vi "Initialize.vi"(7 "Serial Configuration":T1={"Baud Rate"=9600, "Parity"=2, "Data Bits"=7, "Stop Bits"=10, "Flow Control"=0} {"Flow Control" items=["None", "XON/XOFF", "RTS/CTS", "XON/XOFF & RTS/CTS", "DTR/DSR", "XON/XOFF & DTR/DSR"]; "Stop Bits" items=["1.0"=10, "1.5"=15, "2.0"=20]; "Data Bits" items=["7"=7, "8"=8]; "Parity" items=["None", "Odd", "Even", "Mark", "Space"]; "Baud Rate" items=["300"=300, "600"=600, "1200"=1200, "2400"=2400, "4800"=4800, "9600"=9600, "19200"=19200]}, 8 "error in (no error)":errorcluster, 10 "ID Query (False)":bool, 11 "VISA resource name":refnum<visa-resource-name>) -> (0 "error out":errorcluster, 3 "VISA resource name out":refnum<visa-resource-name>)   [LabVIEW 2018]
doc: "Establishes communication with the instrument and optionally performs an instrument identification query and/or an instrument reset. It also places the instrument in a default state needed for other instrument driver operations. Therefore, call this VI before calling other instrument driver VIs for this instrument. Generally, you need to call the <b>Initialize</b> VI only once at the beginning of an application."
panel:
  # "(c) 2014 <Enter Company Name Here>.  ALL RIGHTS RESERVED."
  # "EDIT: Change control description to remove example text for buses not supported."
  # "EDIT: Serial settings must match those on the physical instrument.  Review user's manual to determine the correct Flow Control protocol for the instrument.  \"None\" is the least robust option for this setting, and could lead to unreliable data transmission."
  # "EDIT: If your instrument does not support ID query or Reset, remove the ID Query or Reset control from the front panel and delete the case structure with the ID Query or Reset code from the block diagram."
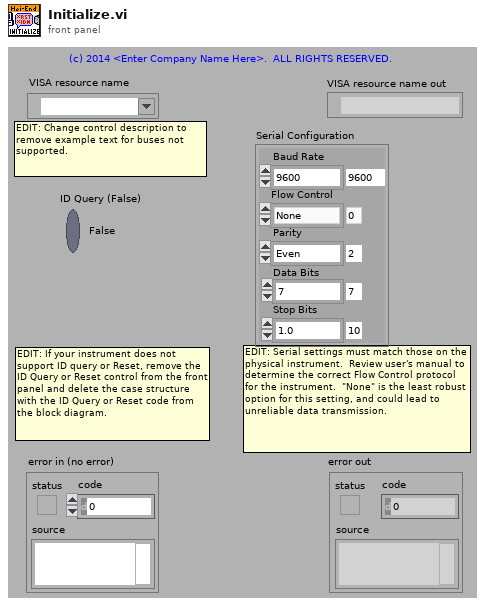
[diagram p1: front panel]
types:
  T1 = cluster{"Baud Rate":u32, "Parity":u16, "Data Bits":u16, "Stop Bits":u16, "Flow Control":u16}
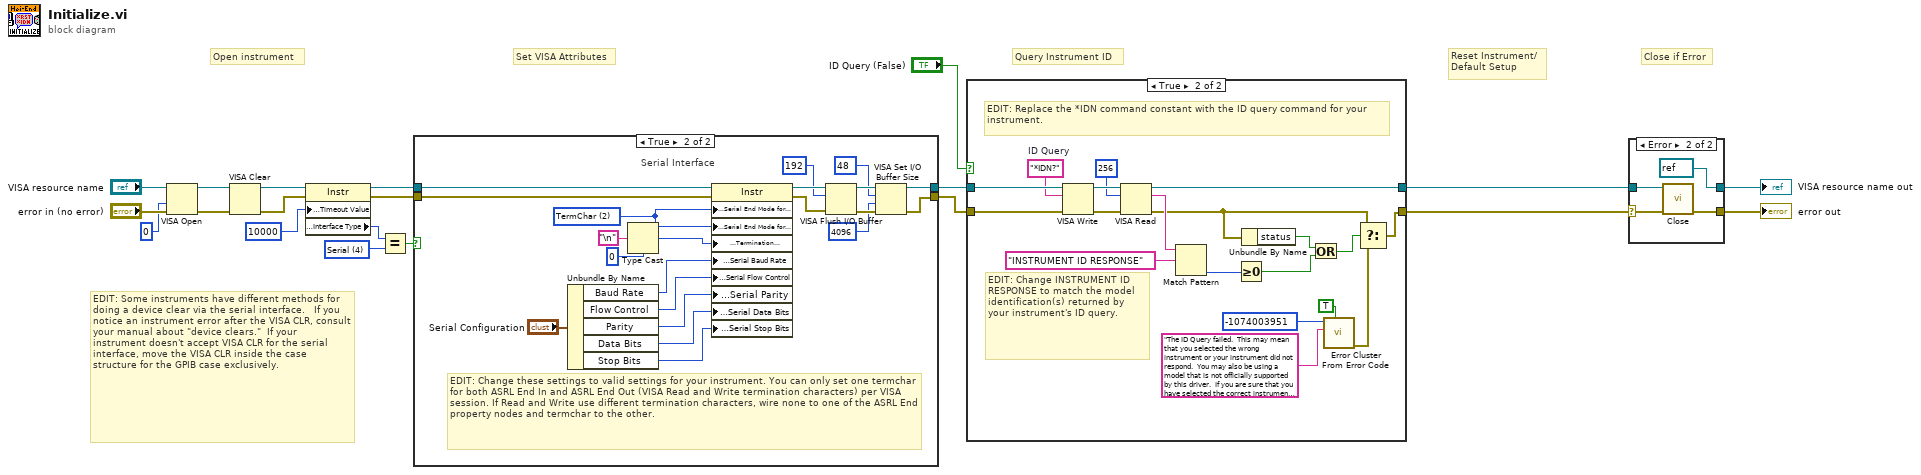
[diagram p0: block diagram]
diagram:
  w10 = u16 4 items=["GPIB"=1, "VXI"=2, "GPIB-VXI"=3, "Serial"=4, "PXI"=5, "TCPIP"=6, "USB"=7] ("Interface Information:Interface Type")
  # "EDIT: Some instruments have different methods for doing a device clear via the serial interface.   If you notice an instrument error after the VISA CLR, consult your manual about \"device clears.\"  If your instrument doesn't accept VISA CLR for the serial interface, move the VISA CLR inside the case  structure for the GPIB case exclusively."
  # "Set VISA Attributes"
  # "Close if Error"
  # "Query Instrument ID"
  # "Reset Instrument/\nDefault Setup"
  # "Open instrument"
  n1 = VISA Open(access mode=u32 0, error in (no error)="error in (no error)", VISA resource name="VISA resource name") -> (VISA resource name=w8:refnum<visa-resource-name>, error out=w7:errorcluster)  [unwired: 2 in]
  n2 = VISA Clear(VISA resource name=w8, error in (no error)=w7) -> (VISA resource name out=w6:refnum<visa-resource-name>, error out=w5:errorcluster)
  n3 = property class="Instr"(reference=w6, error in=w5, "General Settings:Timeout Value"=u32 10000) -> (reference out=w13:refnum<visa-resource-name>, error out=w12:errorcluster, "Interface Information:Interface Type"=w17:u16)
  n4 = Equal?(x=w17, y=w10) -> (x = y?=w11:bool)
  n5 = case shown="True" w11 {
    tunnel: [w21 w40] -> w15
    tunnel: [w22 w37] -> w14
    tunnel: w13 -> [w21 w42]
    tunnel: w12 -> [w22 w43]
    frame False {
      # "EDIT: Remove interfaces not supported by your instrument."
      # "GPIB, TCP/IP, and USB Interface"
    }
    frame True {
      w30 = u16 2 items=["None", "LastBit", "TermChar"] ("Serial Settings:Serial End Mode for Reads")
      # "EDIT: Change these settings to valid settings for your instrument. You can only set one termchar for both ASRL End In and ASRL End Out (VISA Read and Write termination characters) per VISA session. If Read and Write use different termination characters, wire none to one of the ASRL End property nodes and termchar to the other."
      # "Serial Interface"
      n6 = Unbundle By Name("Serial Configuration") -> ("Baud Rate"=w28:u32, "Flow Control"=w24:u16, "Parity"=w26:u16, "Data Bits"=w27:u16, "Stop Bits"=w23:u16)
      n7 = Type Cast(type=u8 0, x="\n" ("Line Feed Constant")) -> (*(type *) &x=w29:u8)
      n8 = property class="Instr"(reference=w42, error in=w43, "Serial Settings:Serial End Mode for Reads"=w30, "Serial Settings:Serial End Mode for Writes"=w30, "Message Based Settings:Termination Character"=w29, "Serial Settings:Serial Baud Rate"=w28, "Serial Settings:Serial Flow Control"=w24, "Serial Settings:Serial Parity"=w26, "Serial Settings:Serial Data Bits"=w27, "Serial Settings:Serial Stop Bits"=w23) -> (reference out=w36:refnum<visa-resource-name>, error out=w39:errorcluster)
      n9 = VISA Flush I/O Buffer(VISA resource name=w36, mask (16)=u16 192, error in (no error)=w39) -> (VISA resource name out=w41:refnum<visa-resource-name>, error out=w38:errorcluster)
      n10 = VISA Set I/O Buffer Size(VISA resource name=w41, mask (16)=u16 48, size (4096)=u32 4096 ("size (0)"), error in (no error)=w38) -> (VISA resource name out=w40:refnum<visa-resource-name>, error out=w37:errorcluster)
    }
  }
  n11 = case shown="True" "ID Query (False)" {
    tunnel: [w44 w64] -> w1
    tunnel: [w45 w61] -> w2
    tunnel: w15 -> [w45 w62]
    tunnel: w14 -> [w44 w63]
    frame False {
    }
    frame True {
      w55 = "*IDN?"  # ID Query
      # "EDIT: Replace the *IDN command constant with the ID query command for your instrument."
      # "EDIT: Change INSTRUMENT ID RESPONSE to match the model identification(s) returned by your instrument's ID query."
      n12 = VISA Write(VISA resource name=w62, write buffer=w55, error in (no error)=w63) -> (VISA resource name out=w59:refnum<visa-resource-name>, error out=w58:errorcluster)  [unwired: 1 out]
      n13 = VISA Read(VISA resource name=w59, byte count=u32 256, error in (no error)=w58) -> (VISA resource name out=w61:refnum<visa-resource-name>, read buffer=w60:string, error out=w49:errorcluster)  [unwired: 1 out]
      n14 = Match Pattern(string=w60, regular expression="INSTRUMENT ID RESPONSE") -> (offset past match=w50:i32)  [unwired: 1 in, 3 out]
      n15 = Greater Or Equal To 0?(x=w50) -> (x >= 0?=w47:bool)
      n16 = Unbundle By Name(w49) -> ("status"=w48:bool)
      n17 = Or(x=w48, y=w47) -> (x .or. y?=w46:bool)
      n18 = call <vilib>:"Error Cluster From Error Code.vi"("show call chain? (False)"=TRUE, "error message (\"\")"="The ID Query failed.  This may mean that you selected the wrong instrument or your instrument did not respond.  You may also be using a model that is not officially supported by this driver.  If you are sure that you have selected the correct instrument and it is responding, try disabling the ID Query." ("Source (VI Name)"), "error code (0)"=-1074003951 ("Code")) -> ("error out"=w54:errorcluster)  [unwired: 6 in]
      n19 = Select(t=w49, s=w46, f=w54) -> (s? t:f=w64:errorcluster)
    }
  }
  n20 = case shown="Error" w1 {
    selector: w1 -> [w66 w69]
    tunnel: [w65 refnum<visa-resource-name> refnum ("VISA resource name out")] -> w4
    tunnel: [w66 w70] -> w3
    tunnel: w2 -> [w65 w67]
    frame No Error {
    }
    frame Error {
      n21 = call "Close.vi"("error in (no error)"=w69, "VISA resource name"=w67) -> ("error out"=w70:errorcluster)  [unwired: 9 in]
    }
  }
  "VISA resource name out" <- w4
  "error out" <- w3
